vi "LVClasse_HasoConfig ctor.vi"(0 "HasoConfig (const)":refnum<class "HasoConfig.lvclass">, 5 "HasoSetupFile":path, 11 "error in (no error)":errorcluster) -> (4 "HasoConfig (new)":refnum<class "HasoConfig.lvclass">, 15 "error out":errorcluster)   [LabVIEW 2020, in "HasoConfig.lvclass"]
doc: "Surface constructor from dimensions and steps.\n\n--------------------------------------------------------------------------------\n\n<B>SurfaceIn </B> : Constant Pointer to Surface object.\n<B>SurfaceOut </B> : Constant Pointer to Surface object.\n<B>dimensions </B> : Surface dimensions (width, height).\n<B>step </B> : Physical step x and y between the surface elements (um).\n<B>ErrorIn </B> : Error\n<B>ErrorOut </B> : Error\n\n--------------------------------------------------------------------------------"
uses:
  HasoConfig.lvclass
  Controls/Handle creation.ctl
  HasoConfig.lvclass/HasoConfig.ctl
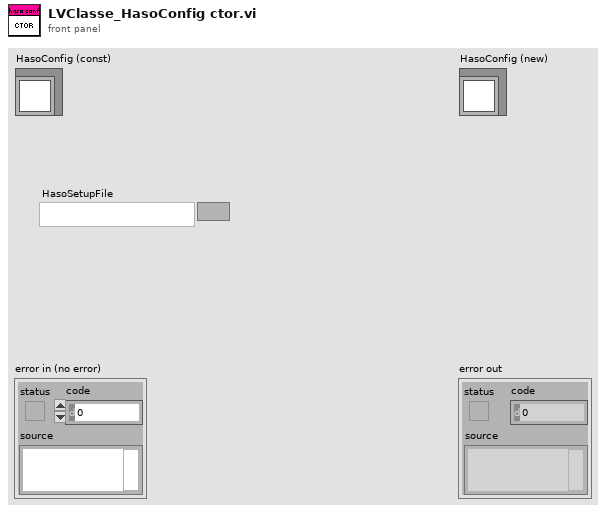
[diagram p1: front panel]
types:
  T1 = typedef "Handle creation.ctl" = enum16{"By ctor", "By write function"}
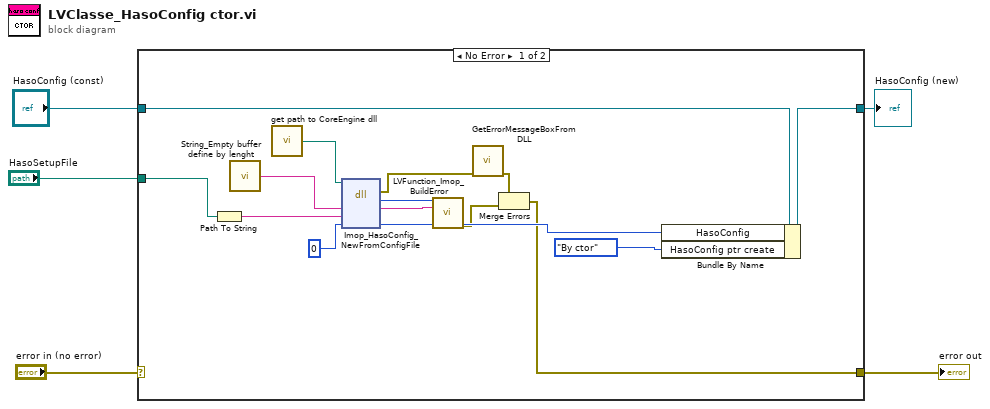
[diagram p0: block diagram]
diagram:
  n1 = case shown="No Error" "error in (no error)" {
    selector: "error in (no error)" -> [_ w22]
    tunnel: [w8 w22] -> w4
    tunnel: [w12 w21] -> w2
    tunnel: "HasoConfig (const)" -> [w13 w21]
    tunnel: "HasoSetupFile" -> [w7 _]
    frame No Error {
      n2 = Path To String(path=w7) -> (string=w6:string)
      n3 = call "String_Empty buffer define by lenght.vi"() -> ("Empty buffer"=w17:string)  [unwired: 1 in]
      n4 = call "get path to CoreEngine dll.vi"() -> ("path to wavekit library"=w16:path)  [unwired: 14 in, 1 out]
      n5 = dll-call lib="D:/soft/HASO_v3/SVN_trunk/ImOpCoreEngine4_LV2011/DLLs/c_interface_vc100.dll" fn="Imop_HasoConfig_NewFromConfigFile"(path in=w16, "message"=w17, "HasoSetupFile"=w6, "HasoConfig"=0 ("objet")) -> (error out=w11:errorcluster, "return type"=w20:i32, "message"=w19:string, "HasoConfig"=w18:i64)  [unwired: 3 in, 1 out]
      n6 = call "LVFunction_Imop_BuildError.vi"("code"=w20, "String to Prepend to source (\"\")"=w19) -> ("error out"=w9:errorcluster)  [unwired: 13 in]
      n7 = call "GetErrorMessageBoxFromDLL.vi"("error IN"=w11) -> ("error OUT"=w10:errorcluster)  [unwired: 10 in]
      n8 = Merge Errors(w10, w9) -> (w8:errorcluster)
      n9 = Bundle By Name(cluster=w13, "HasoConfig"=w18, "HasoConfig ptr create"=Handle_creation."By ctor" ("HasoData ptr create")) -> (w12:refnum<class "HasoConfig.lvclass">)
    }
    frame Error {
    }
  }
  "error out" <- w4
  "HasoConfig (new)" <- w2
